vi "Initialize.vi"(8 "error in (no error)":errorcluster, 11 "VISA Reference":refnum<visa-resource-name>) -> (0 "error out":errorcluster, 3 "dup VISA resource name":refnum<visa-resource-name>)   [LabVIEW 2016]
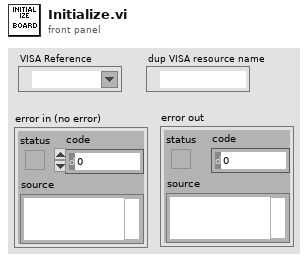
[diagram p1: front panel]
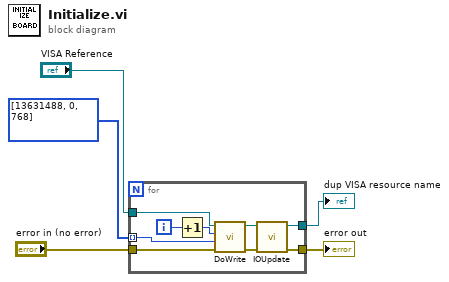
[diagram p0: block diagram]
diagram:
  n1 = for {
    tunnel: "VISA Reference" -> [w12]
    tunnel: "error in (no error)" -> [w11]
    tunnel: [w9] -> w5
    tunnel: [w10] -> w4
    tunnel: i32[] [13631488, 0, 768] -> [w8] mode=indexing
    i -> [w7]
    n2 = Increment(x=w7) -> (x+1=w6:i32)
    n3 = call "DoWrite.vi"("error in (no error)"=w11, "Value"=w8, "Register Address"=w6, "VISA Reference"=w12) -> ("error out"=w13:errorcluster, "dup VISA resource name"=w14:refnum<visa-resource-name>)  [unwired: 6 in]
    n4 = call "IOUpdate.vi"("error in (no error)"=w13, "VISA Reference"=w14) -> ("error out"=w9:errorcluster, "dup VISA resource name"=w10:refnum<visa-resource-name>)  [unwired: 8 in]
  }
  "dup VISA resource name" <- w4
  "error out" <- w5
